vi "LogMark10Event.vi"(7 "Type":enum16{"Tx", "Rx"}(ring)=enum."Rx", 8 "Error In":errorcluster, 11 "Event":string) -> (0 "Error Out":errorcluster)   [LabVIEW 2019, in "Mark 10 TSTM-DC.lvlib" / "Mark 10 Event Monitor.lvlib"]
uses:
  Mark 10 Event Monitor.lvlib
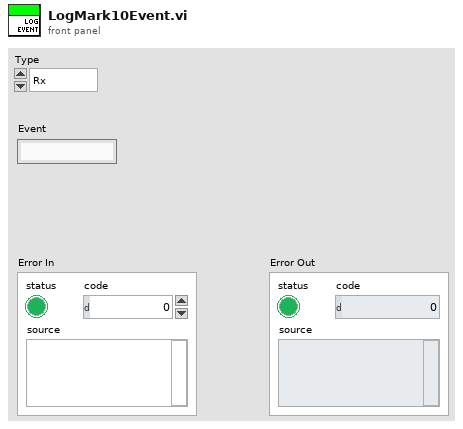
[diagram p1: front panel]
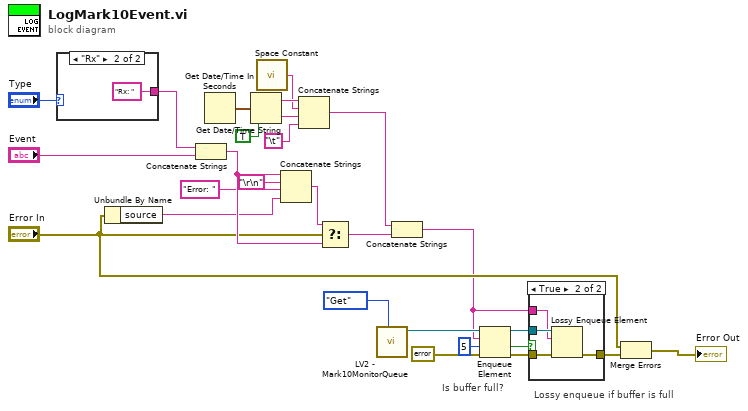
[diagram p0: block diagram]
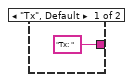
[diagram p3: hidden frame]
diagram:
  # "Lossy enqueue if buffer is full"
  # "Is buffer full?"
  n1 = case shown="\"Rx\"" "Type" {
    tunnel: ["Tx: " ("string") "Rx: " ("string")] -> w22
    frame "Tx", Default {
    }
    frame "Rx" {
    }
  }
  n2 = Unbundle By Name("Error In") -> ("source"=w16:string)
  n3 = Concatenate Strings(w22, "Event") -> (w19:string)
  n4 = Get Date/Time In Seconds() -> (seconds since 1Jan1904=w12:timestamp)
  n5 = Get Date/Time String(seconds (now)=w12, want seconds? (F)=TRUE) -> (date string=w11:string, time string=w10:string)  [unwired: 1 in]
  n6 = call <vilib>:"Space Constant.vi"() -> ("String"=w9:string)
  n7 = Concatenate Strings(w19, "\r\n", "Error: " ("string"), w16) -> (w15:string)
  n8 = Concatenate Strings(w11, w9, w10, "\t") -> (w8:string)
  n9 = Select(t=w15, s="Error In", f=w19) -> (s? t:f=w20:string)
  n10 = call "LV2 - Mark10MonitorQueue.vi"("Enum"=enum16{"Set", "Get"}."Get") -> ("Mark10Monitor out"=w25:refnum<queue>)  [unwired: 10 in]
  n11 = Concatenate Strings(w8, w20) -> (w1:string)
  n12 = Enqueue Element(queue=w25, element=w1, timeout in ms (-1)=5, error in (no error)=errorcluster {"status"=FALSE, "code"=0, "source"=""}) -> (queue out=w3:refnum<queue>, timed out?=w2:bool, error out=w27:errorcluster)
  n13 = case shown="True" w2 {
    tunnel: w27 -> [w30 w34]
    tunnel: [w30 w33] -> w4
    tunnel: w3 -> [_ w32]
    tunnel: w1 -> [_ w31]
    frame False {
    }
    frame True {
      n14 = Lossy Enqueue Element(queue=w32, element=w31, error in (no error)=w34) -> (error out=w33:errorcluster)  [unwired: 3 out]
    }
  }
  n15 = Merge Errors("Error In", w4) -> (→"Error Out":errorcluster)
